vi "post_modification.vi"(8 "error in":errorcluster, 11 "Instrument Command In":string) -> (0 "error out":errorcluster, 3 "Instrument Command Out":string)   [LabVIEW 2018]
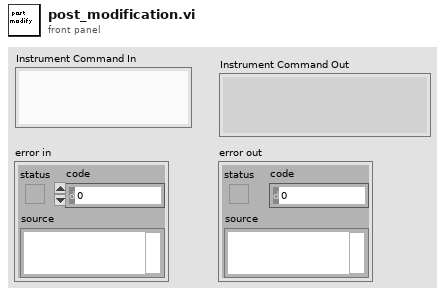
[diagram p1: front panel]
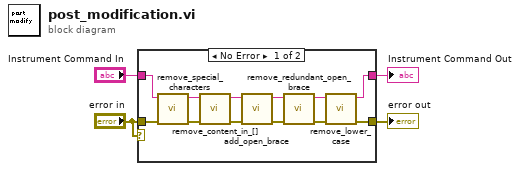
[diagram p0: block diagram]
diagram:
  n1 = case shown="No Error" "error in" {
    tunnel: "Instrument Command In" -> [w16 w18]
    tunnel: "error in" -> [w15 w17]
    tunnel: [w6 w17] -> w3
    tunnel: [w5 w18] -> w2
    frame No Error {
      n2 = call "remove_special_characters.vi"("error in (no error)"=w15, "Instrument Command In"=w16) -> ("error out"=w14:errorcluster, "Instrument Command Out"=w13:string)  [unwired: 8 out]
      n3 = call "remove_content_in_[].vi"("error in (no error)"=w14, "Instrument Command In"=w13) -> ("error out"=w12:errorcluster, "Instrument Command Out"=w11:string)  [unwired: 8 out]
      n4 = call "add_open_brace.vi"("error in (no error)"=w12, "Instrument Command In"=w11) -> ("error out"=w10:errorcluster, "Instrument Command Out"=w9:string)  [unwired: 8 out]
      n5 = call "remove_redundant_open_brace.vi"("error in (no error)"=w10, "Instrument Command In"=w9) -> ("error out"=w7:errorcluster, "Instrument Command Out"=w8:string)  [unwired: 8 out]
      n6 = call "remove_lower_case.vi"("error in (no error)"=w7, "Instrument Command In"=w8) -> ("error out"=w6:errorcluster, "Instrument Command Out"=w5:string)  [unwired: 8 out]
    }
    frame Error {
    }
  }
  "error out" <- w3
  "Instrument Command Out" <- w2
